vi "Configure Output Delay.vi"(8 "error in (no error)":errorcluster, 9 "Output Turn-Off Sequence Delay (0)":dbl, 10 "Output Turn-On Sequence Delay (0)":dbl, 11 "VISA resource name":refnum<visa-resource-name>) -> (0 "error out":errorcluster, 3 "VISA resource name out":refnum<visa-resource-name>)   [LabVIEW 2019, in "Agilent N7976A.lvlib"]
doc: "Configures the delay in seconds that the instrument waits before turning the output on (rise) or off (fall). This allows multiple instruments to turn on or off in sequence."
uses:
  <instrlib>/Agilent N7976A/Agilent N7976A.lvlib
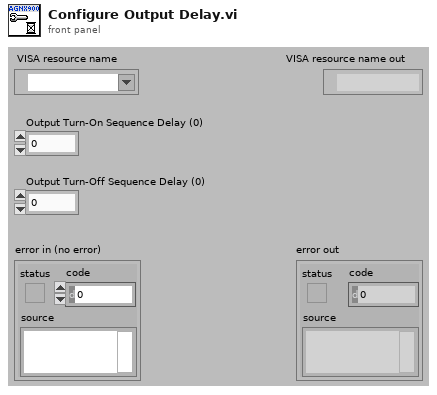
[diagram p1: front panel]
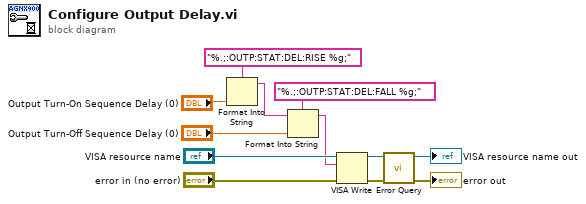
[diagram p0: block diagram]
diagram:
  n1 = Format Into String(format string="%.;:OUTP:STAT:DEL:RISE %g;", "Output Turn-On Sequence Delay (0)") -> (resulting string=w3:string)  [unwired: 2 in, 1 out]
  n2 = Format Into String(format string="%.;:OUTP:STAT:DEL:FALL %g;", initial string=w3, "Output Turn-Off Sequence Delay (0)") -> (resulting string=w6:string)  [unwired: 1 in, 1 out]
  n3 = VISA Write(VISA resource name="VISA resource name", write buffer=w6, error in (no error)="error in (no error)") -> (VISA resource name out=w9:refnum<visa-resource-name>, error out=w10:errorcluster)  [unwired: 1 out]
  n4 = call <instrlib>:"Error Query.vi"("error in (no error)"=w10, "VISA resource name"=w9) -> ("error out"=→"error out":errorcluster, "VISA resource name out"=→"VISA resource name out":refnum<visa-resource-name>)  [unwired: 6 in, 2 out]
